vi "Plot X-Y with names.vi"(6 "Set axes names":bool=TRUE, 8 "Error In":errorcluster, 9 "Y columns":waveform(dbl)[](array[waveform]), 10 "X column":waveform(dbl), 11 "XY Graph Ref":refnum<vi>) -> (0 "Error Out":errorcluster, 3 "XYGraph Refnum out":refnum<vi>)   [LabVIEW 2015]
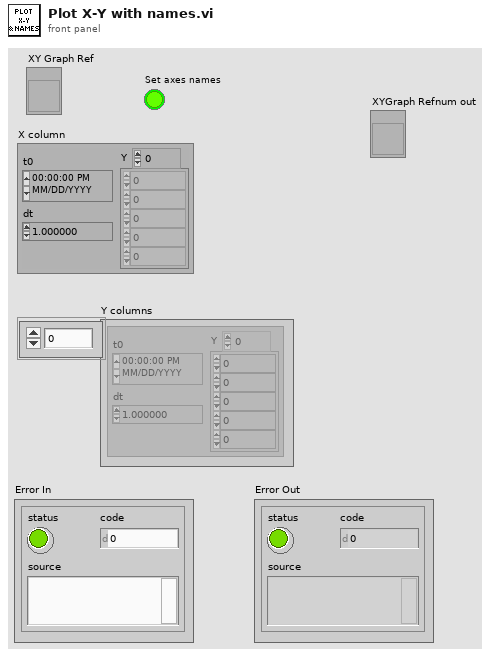
[diagram p1: front panel]
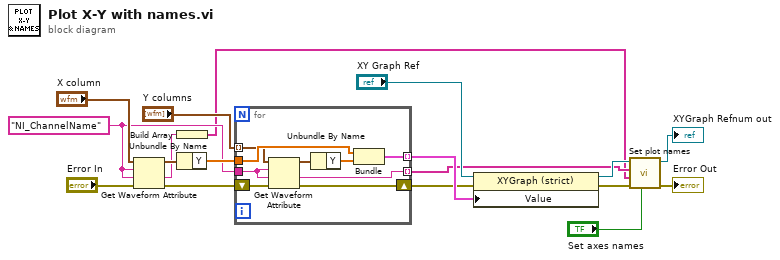
[diagram p0: block diagram]
diagram:
  w10 = "NI_ChannelName" ("name")
  n1 = Get Waveform Attribute(4:"Error In", 5:w10, 6:w10, 7:"X column") -> (0:w8:errorcluster, 1:w6:string, 3:w7:waveform(dbl))  [unwired: 1 out]
  n2 = Build Array(w6) -> (w5:string[])
  n3 = Unbundle By Name(w7) -> ("Y"=w18:dbl[])
  n4 = for {
    tunnel: "Y columns" -> [w24] mode=indexing
    tunnel: w18 -> [w27]
    tunnel: [w26] -> w15 mode=indexing
    shift-right: [w22] -> w9
    shift-left: w8 -> [w23]
    tunnel: w10 -> [w21]
    tunnel: [w20] -> w12 mode=indexing
    n5 = Get Waveform Attribute(4:w23, 5:w21, 6:w21, 7:w24) -> (0:w22:errorcluster, 1:w20:string, 3:w19:waveform(dbl))  [unwired: 1 out]
    n6 = Unbundle By Name(w19) -> ("Y"=w25:dbl[])
    n7 = Bundle("Y"=w27, "Y"=w25) -> (w26:cluster{"Y":dbl[], "Y":dbl[]})  [unwired: 1 out]
  }
  n8 = property class="XYGraph (strict)"(reference="XY Graph Ref", error in=w9, "Value"=w15) -> (reference out=w14:refnum<vi>, error out=w13:errorcluster)
  n9 = call "Set plot names.vi"("Set axes names"="Set axes names", "error in"=w13, "X-axis names"=w5, "Plot names"=w12, "XYGraph Refnum"=w14) -> ("error out"=→"Error Out":errorcluster, "XYGraph Refnum out"=→"XYGraph Refnum out":refnum<vi>)  [unwired: 5 in]
